vi "扭矩.vi"   [LabVIEW 2020]
uses:
  <userlib>/DAQNavi Polymorphic VI/create/DAQNavi Create Channel(AI-Voltage).vi
  Global_Variable/Global.vi
  Global_Variable/A131258.vi
  <userlib>/DAQNavi Polymorphic VI/read/DAQNavi Read (Analog 1D DBL NChan 1Samp).vi
  <userlib>/_MGI/1D Array/MGI Running Average/MGI Running Average(DBL).vi
  <vilib>/ptbypt/NI_PtbyPt.lvlib
types:
  T1 = cluster{"左平均扭矩":cluster{"正转":dbl, "反转":dbl}, "左矩波动":cluster{"正转":dbl, "反转":dbl}, "左空载":cluster{"正转":dbl, "反转":dbl}, "右平均扭矩":cluster{"正转":dbl, "反转":dbl}, "右扭矩波动":cluster{"正转":dbl, "反转":dbl}, "右空载":cluster{"正转":dbl, "反转":dbl}, "扭矩对称":cluster{"左":dbl, "右":dbl}, "左零点漂移":cluster{"正":dbl, "反":dbl}, "右零点漂移":cluster{"正":dbl, "反":dbl}}
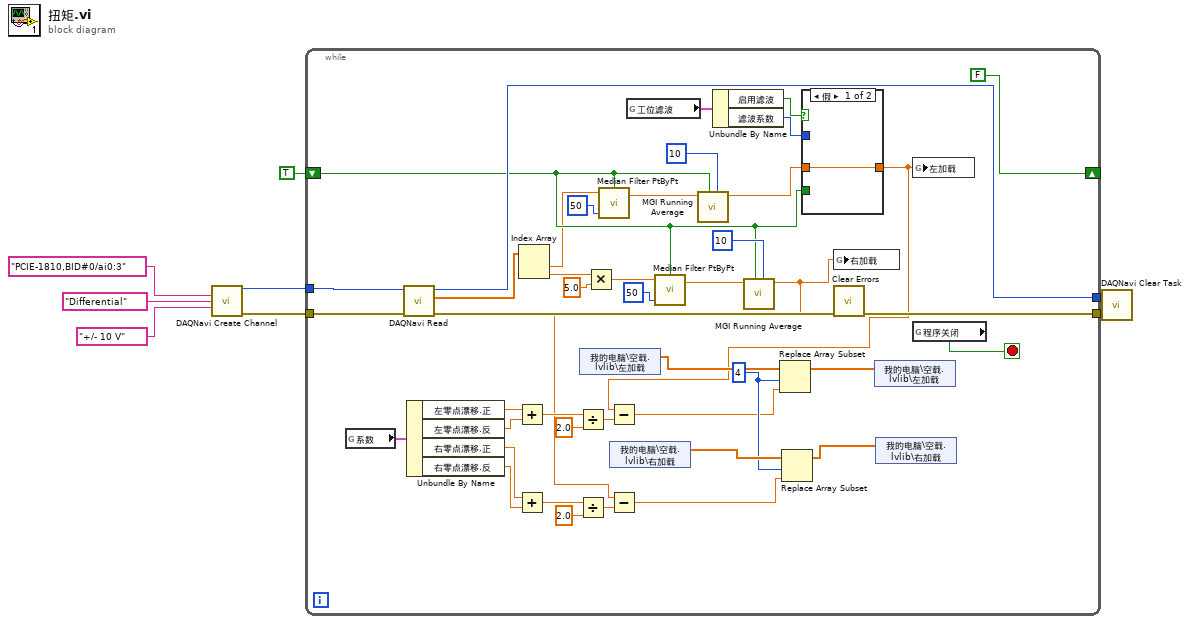
[diagram p0: block diagram]
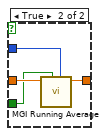
[diagram p2: hidden frame]
diagram:
  n1 = call-poly <userlib>:"DAQNavi Create Channel.vi"("physical channels"="PCIE-1810,BID#0/ai0:3", "signal type"="Differential", "value range"="+/- 10 V") -> ("task out"=w6:i32, "error out"=w5:errorcluster)  [unwired: 11 in]
  n2 = while {
    tunnel: w6 -> [w51]
    tunnel: w5 -> [w50]
    tunnel: [w46] -> w3
    tunnel: [w47] -> w2
    shift-right: [FALSE] -> _
    shift-left: TRUE -> [w34]
    stop <- w49 stop-if-true
    w25 = 4 ("索引")
    n3 = global read "A131258.vi" "系数"() -> (w13:T1)
    n4 = call-poly <userlib>:"DAQNavi Read.vi"("error in (no error)"=w50, "task in"=w51) -> ("error out"=w48:errorcluster, "data"=w45:dbl[], "task out"=w47:i32)  [unwired: 7 in]
    n5 = Unbundle By Name(w13) -> ("左零点漂移.正"=w14:dbl, "左零点漂移.反"=w15:dbl, "右零点漂移.正"=w20:dbl, "右零点漂移.反"=w21:dbl)
    n6 = Add(x=w14, y=w15) -> (x+y=w16:dbl)
    n7 = Add(x=w20, y=w21) -> (x+y=w19:dbl)
    n8 = Index Array(array=w45) -> (element #1=w32:dbl, element #2=w31:dbl)  [unwired: 2 in]
    n9 = Divide(x=w16, y=2.0) -> (x/y=w17:dbl)
    n10 = Divide(x=w19, y=2.0) -> (x/y=w18:dbl)
    n11 = shared-variable "我的电脑\\空载.lvlib\\左加载"() -> (w28:sgl[])  [unwired: 1 in, 1 out]
    n12 = Multiply(x=w31, y=5.0) -> (x*y=w30:dbl)
    n13 = call <vilib>:"Median Filter PtByPt.vi"("initialize"=w34, "rank"=50, "x"=w32) -> ("Filtered x"=w43:dbl)  [unwired: 1 in, 1 out]
    n14 = shared-variable "我的电脑\\空载.lvlib\\右加载"() -> (w26:sgl[])  [unwired: 1 in, 1 out]
    n15 = global read "A131258.vi" "工位滤波"() -> (w37:cluster{"启用滤波":bool, "滤波系数":i8})
    n16 = call <vilib>:"Median Filter PtByPt.vi"("initialize"=w34, "rank"=50, "x"=w30) -> ("Filtered x"=w44:dbl)  [unwired: 1 in, 1 out]
    n17 = call-poly <userlib>:"MGI Running Average.vi"("Averaging Size"=10, "Initialize? (F)"=w34, "Value"=w43) -> ("Average"=w35:dbl)  [unwired: 8 in]
    n18 = Unbundle By Name(w37) -> ("启用滤波"=w36:bool, "滤波系数"=w33:i8)
    n19 = call-poly <userlib>:"MGI Running Average.vi"("Averaging Size"=10, "Initialize? (F)"=w34, "Value"=w44) -> ("Average"=w9:dbl)  [unwired: 8 in]
    n20 = Subtract(x=w9, y=w18) -> (x-y=w11:dbl)
    n21 = Replace Array Subset(array=w26, new element=w11, index=w25) -> (w24:sgl[])
    n22 = case shown="假" w36 {
      tunnel: w35 -> [w52 w56]
      tunnel: w34 -> [_ w55]
      tunnel: w33 -> [_ w54]
      tunnel: [w52 w53] -> w10
      frame False {
      }
      frame True {
        n23 = call-poly <userlib>:"MGI Running Average.vi"("Averaging Size"=w54, "Initialize? (F)"=w55, "Value"=w56) -> ("Average"=w53:dbl)  [unwired: 8 in]
      }
    }
    n24 = Subtract(x=w10, y=w17) -> (x-y=w12:dbl)
    n25 = Replace Array Subset(array=w28, new element=w12, index=w25) -> (w27:sgl[])
    n26 = global write "全局2.vi" "右加载"(w9) -> ()
    n27 = call <vilib>:"Clear Errors.vi"("error in (no error)"=w48) -> ("error out"=w46:errorcluster)  [unwired: 5 in, 1 out]
    n28 = shared-variable "我的电脑\\空载.lvlib\\左加载"(w27) -> ()  [unwired: 1 in, 1 out]
    n29 = shared-variable "我的电脑\\空载.lvlib\\右加载"(w24) -> ()  [unwired: 1 in, 1 out]
    n30 = global write "全局1.vi" "左加载"(w10) -> ()
    n31 = global read "Global.vi" "程序关闭"() -> (w49:bool)
  }
  n32 = call <userlib>:"DAQNavi Clear Task.vi"("error in (no error)"=w3, "task in"=w2) -> ()  [unwired: 1 in, 1 out]
